vi "Identify Response.vi"(8 "error in":errorcluster, 10 "Input String":string) -> (0 "error out":errorcluster, 2 "Is SMS Response":bool)   [LabVIEW 2025]
doc: "Checks if the input string matches the expected format of the SMS power supply's reponse to an identification query."
uses:
  <vilib>/regexp/Match Regular Expression.xnode
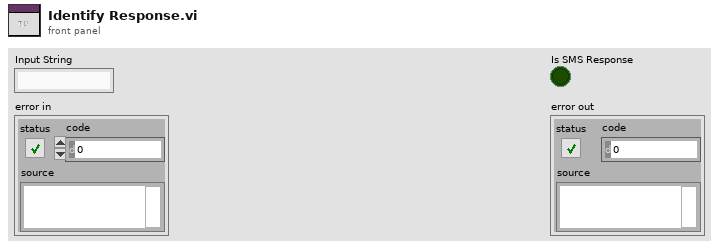
[diagram p1: front panel]
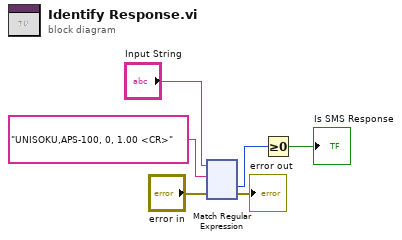
[diagram p0: block diagram]
diagram:
  n1 = xnode "Match Regular Expression"("input string"="Input String", "regular expression"="UNISOKU,APS-100, 0, 1.00 <CR>", "error in"="error in") -> ("offset past match"=w6:i32, "error out"=→"error out":errorcluster)  [unwired: 3 in, 3 out]
  n2 = Greater Or Equal To 0?(x=w6) -> (x >= 0?=→"Is SMS Response":bool)
